vi "VCS Reset Port Name Selection.vi"(0 "device in":T1={"deviceName"="EPOS2", "protocolStackName"="MAXON SERIAL V2", "interfaceName"="USB"}, 11 "error in (no error)":errorcluster) -> (4 "device out":T1={"deviceName"="EPOS2", "protocolStackName"="MAXON SERIAL V2", "interfaceName"="USB"}, 15 "error out":errorcluster)   [LabVIEW 2019, in "maxonEPOS.lvlib"]
doc: "<B>VCS Get Port Name Selection</B> returns all available port names."
uses:
  Examples/maxonEPOS.lvlib
  Resources/EposCmd.dll
  Resources/EposCmd64.dll
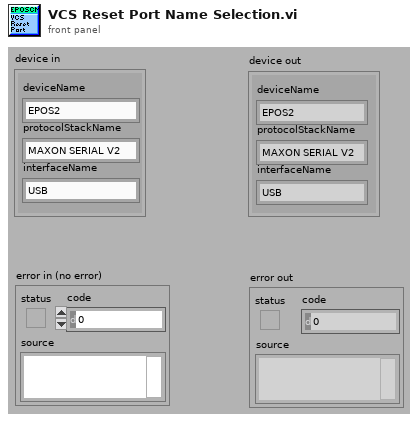
[diagram p1: front panel]
types:
  T1 = cluster{"deviceName":string, "protocolStackName":string, "interfaceName":string}
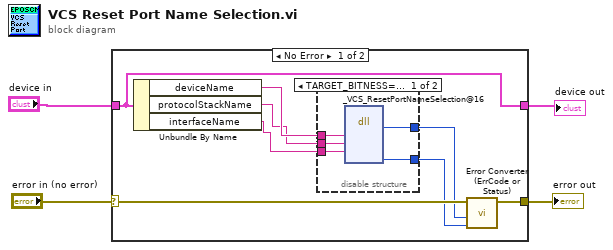
[diagram p0: block diagram]
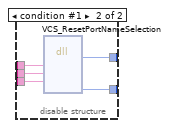
[diagram p2: hidden frame]
diagram:
  n1 = case shown="No Error" "error in (no error)" {
    selector: "error in (no error)" -> [w12 w24]
    tunnel: [w11 w24] -> w3
    tunnel: "device in" -> [w7 w23]
    tunnel: [w7 w23] -> w1
    frame No Error {
      n2 = Unbundle By Name(w7) -> ("deviceName"=w10:string, "protocolStackName"=w9:string, "interfaceName"=w8:string)
      n3 = disable-structure shown="TARGET_BITNESS==32, Standard" {
        disable-tunnel: w10 -> [w17 w22]
        disable-tunnel: w9 -> [w16 w21]
        disable-tunnel: w8 -> [w15 w20]
        disable-tunnel: [w14 w19] -> w6
        disable-tunnel: [w13 w18] -> w5
        frame condition #0 (active) {
          n4 = dll-call lib="C:/workspace/project/scancon/sw/SSI_Tool/InstrumentsInterfaces/Motordriver/maxon EPOS/Resources/EposCmd.dll" fn="_VCS_ResetPortNameSelection@16"("DeviceName"=w17, "ProtocolStackName"=w16, "InterfaceName"=w15) -> (w14:i32, "pErrorCode"=w13:u32)  [unwired: 7 in, 2 out]
        }
        frame condition #1 {
          n5 = dll-call lib="C:/setup/Resources/EposCmd64.dll" fn="VCS_ResetPortNameSelection"("DeviceName"=w22, "ProtocolStackName"=w21, "InterfaceName"=w20) -> ("Rückgabetyp"=w19:i32, "pErrorCode"=w18:u32)  [unwired: 7 in, 2 out]
        }
      }
      n6 = call "Error Converter (ErrCode or Status).vi"("error code"=w5, "return type"=w6, "error in (no error)"=w12) -> ("error out"=w11:errorcluster)  [unwired: 7 in]
    }
    frame Error {
    }
  }
  "error out" <- w3
  "device out" <- w1
